vi "Array generation.vi"() -> ()   [LabVIEW 2012]
panel:
  out "deleted portion":dbl[](array[numeric])
  out "array w/ subset deleted":dbl[][](array[numeric])
  out "insert array":dbl[][](array[numeric])
  out "replaced array row replaced":dbl[][](array[numeric])
  out "replace array replaced element":dbl[][](array[numeric])
  out "element":dbl
  out "subarray":dbl[](array[numeric])
  out "size(s)":i32[](array[numeric])
  out "Main Array":dbl[][](array[numeric])
  # "no. of rows"
  # "no. of columns"
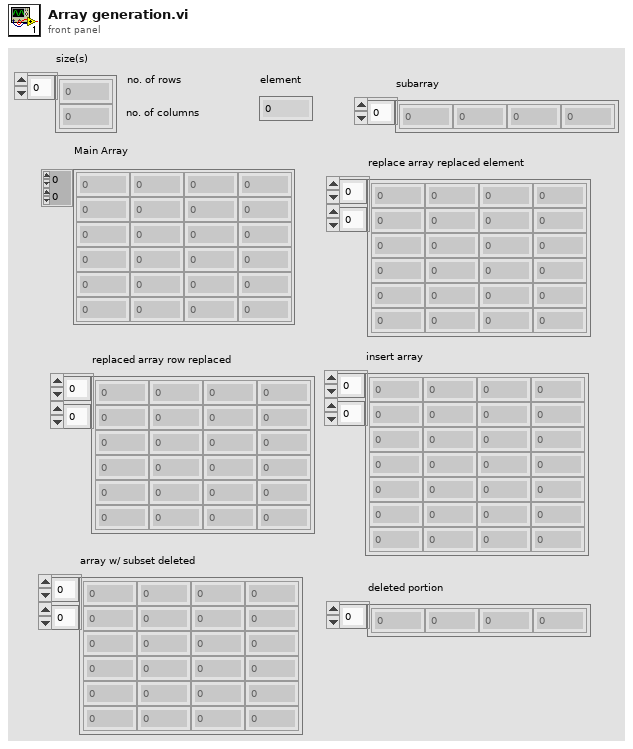
[diagram p1: front panel]
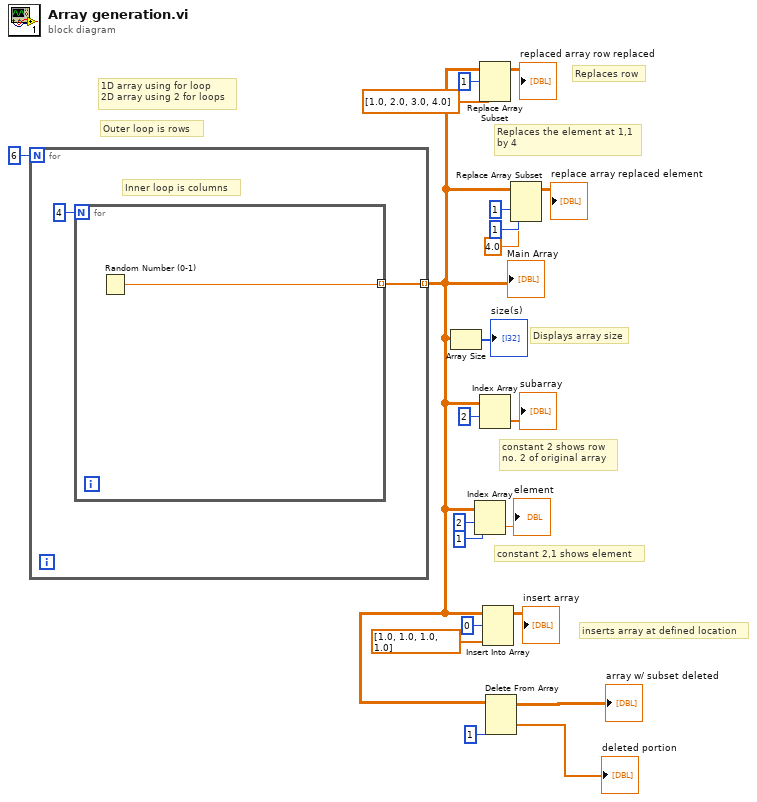
[diagram p0: block diagram]
diagram:
  # "inserts array at defined location"
  # "Replaces row"
  # "Replaces the element at 1,1\nby 4"
  # "1D array using for loop\n2D array using 2 for loops"
  # "constant 2,1 shows element"
  # "constant 2 shows row\nno. 2 of original array"
  # "Displays array size"
  # "Outer loop is rows"
  n1 = for {
    N: 6 -> [_]
    tunnel: [w23] -> w4 mode=indexing
    # "Inner loop is columns"
    n2 = for {
      N: 4 -> [_]
      tunnel: [w24] -> w23 mode=indexing
      n3 = Random Number (0-1)() -> (number: 0 to 1=w24:dbl)
    }
  }
  "Main Array" <- w4
  n4 = Array Size(array=w4) -> (size(s)=→"size(s)":i32[])
  n5 = Index Array(array=w4, index (row)=2, index (col)=1 ("disabled index (col)")) -> (element=→"element":dbl)
  n6 = Replace Array Subset(array=w4, new element=dbl[] [1.0, 2.0, 3.0, 4.0] ("new element/subarray"), index (row)=1) -> (→"replaced array row replaced":dbl[][])  [unwired: 1 in]
  n7 = Index Array(array=w4, index (row)=2) -> (element=→"subarray":dbl[])  [unwired: 1 in]
  n8 = Insert Into Array(array=w4, index (row)=0, new element=dbl[] [1.0, 1.0, 1.0, 1.0] ("new element/subarray")) -> (→"insert array":dbl[][])  [unwired: 1 in]
  n9 = Delete From Array(array=w4, index (row)=1) -> (deleted portion=→"deleted portion":dbl[], array with subset deleted=→"array w/ subset deleted":dbl[][])  [unwired: 2 in]
  n10 = Replace Array Subset(array=w4, new element=4.0 ("new element/subarray"), index (row)=1 ("disabled index (row)"), index (col)=1 ("disabled index (col)")) -> (→"replace array replaced element":dbl[][])
